vi "Controllers_PIDoff.vi"(6 "DC Bias":dbl, 8 "Error In":errorcluster, 11 "Task in":refnum<k21>) -> (0 "Error Out":errorcluster, 3 "Task Out":refnum<k21>)   [LabVIEW 2023]
uses:
  <vilib>/DAQmx/write.llb/DAQmx Write (Analog 1D DBL NChan 1Samp).vi
  <vilib>/DAQmx/miscellaneous.llb/DAQmx Fill In Error Info.vi
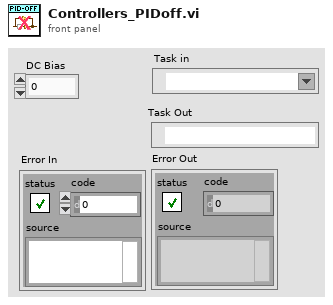
[diagram p1: front panel]
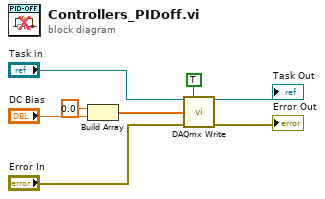
[diagram p0: block diagram]
diagram:
  n1 = Build Array(0.0 ("element"), "DC Bias") -> (w2:dbl[])
  n2 = call-poly <vilib>:"DAQmx Write.vi"("task/channels in"="Task in", "auto start"=TRUE, "data"=w2, "error in"="Error In") -> ("task out"=→"Task Out":refnum<k21>, "error out"=→"Error Out":errorcluster)  [unwired: 9 in, 1 out]
